vi "remove_special_characters.vi"(8 "error in (no error)":errorcluster, 11 "Instrument Command In":string) -> (0 "error out":errorcluster, 3 "Instrument Command Out":string)   [LabVIEW 2018]
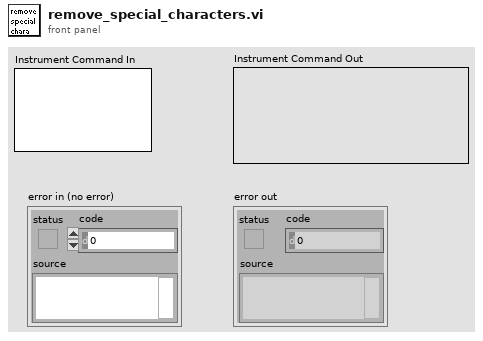
[diagram p1: front panel]
types:
  T1 = cluster{"Start Sting":string, "End String":string}
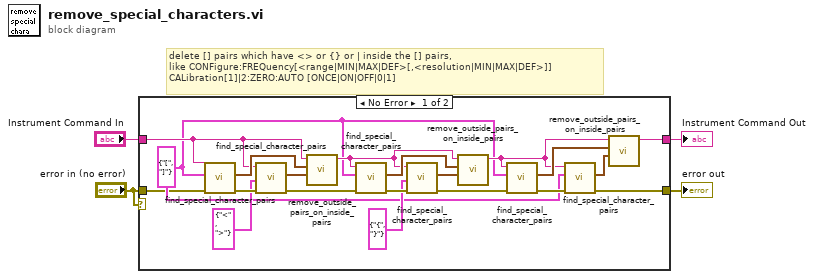
[diagram p0: block diagram]
diagram:
  # "delete [] pairs which have <> or {} or | inside the [] pairs, \nlike CONFigure:FREQuency[<range|MIN|MAX|DEF>[,<resolution|MIN|MAX|DEF>]]\nCALibration[1]|2:ZERO:AUTO [ONCE|ON|OFF|0|1]"
  n1 = case shown="No Error" "error in (no error)" {
    tunnel: "Instrument Command In" -> [w15 w25]
    tunnel: "error in (no error)" -> [w5 w26]
    tunnel: [w6 w25] -> w3
    tunnel: [w7 w26] -> w2
    frame No Error {
      w9 = T1 {"Start Sting"="[", "End String"="]"} ("String Pair")
      n2 = call "find_special_character_pairs.vi"("error in (no error)"=w5, "String Pair"=w9, "Command String"=w15) -> ("error out"=w23:errorcluster, "Pair Offset"=w24:cluster{"Start Offset":i32, "End offset":i32}[])  [unwired: 7 out]
      n3 = call "find_special_character_pairs.vi"("error in (no error)"=w23, "String Pair"=T1 {"Start Sting"="<", "End String"=">"}, "Command String"=w15) -> ("error out"=w14:errorcluster, "Pair Offset"=w22:cluster{"Start Offset":i32, "End offset":i32}[])  [unwired: 7 out]
      n4 = call "remove_outside_pairs_on_inside_pairs.vi"("Inside Pair Offset"=w22, "Outside Pair Offset"=w24, "Instrument Command In"=w15) -> ("Instrument Command Out"=w17:string)  [unwired: 8 out]
      n5 = call "find_special_character_pairs.vi"("error in (no error)"=w14, "String Pair"=w9, "Command String"=w17) -> ("error out"=w20:errorcluster, "Pair Offset"=w21:cluster{"Start Offset":i32, "End offset":i32}[])  [unwired: 7 out]
      n6 = call "find_special_character_pairs.vi"("error in (no error)"=w20, "String Pair"=T1 {"Start Sting"="{", "End String"="}"}, "Command String"=w17) -> ("error out"=w8:errorcluster, "Pair Offset"=w19:cluster{"Start Offset":i32, "End offset":i32}[])  [unwired: 7 out]
      n7 = call "remove_outside_pairs_on_inside_pairs.vi"("Inside Pair Offset"=w19, "Outside Pair Offset"=w21, "Instrument Command In"=w17) -> ("Instrument Command Out"=w10:string)  [unwired: 8 out]
      n8 = call "find_special_character_pairs.vi"("error in (no error)"=w8, "String Pair"=w9, "Command String"=w10) -> ("error out"=w12:errorcluster, "Pair Offset"=w11:cluster{"Start Offset":i32, "End offset":i32}[])  [unwired: 7 out]
      n9 = call "find_special_character_pairs.vi"("error in (no error)"=w12, "String Pair"=w9, "Command String"=w10) -> ("error out"=w7:errorcluster, "Pair Offset"=w13:cluster{"Start Offset":i32, "End offset":i32}[])  [unwired: 7 out]
      n10 = call "remove_outside_pairs_on_inside_pairs.vi"("Inside Pair Offset"=w13, "Outside Pair Offset"=w11, "Instrument Command In"=w10) -> ("Instrument Command Out"=w6:string)  [unwired: 8 out]
    }
    frame Error {
    }
  }
  "Instrument Command Out" <- w3
  "error out" <- w2
